vi "Test Pose.vi"() -> ()   [LabVIEW 2020, in "Rover.lvlib" / "Rover.lvclass"]
uses:
  Rover.lvclass
  Pose.ctl
  PID Tuning.ctl
  <vilib>/MakerHub/LINX/Public/Utilities/Open Local.vi
  <vilib>/MakerHub/LINX/LMH-LINX.lvlib
panel:
  out "OutR":i16(slide) scale=-32767.0..32767.0
  out "OutL":i16(slide) scale=-32767.0..32767.0
  out "Fault":bool
  in  "Turn":sgl(slide) scale=3.0..-3.0
  in  "Drive":sgl(slide) scale=-2.0..2.0
  in  "PID Tuning":T1
  out "XY Graph":cluster{"X":dbl, "Y":dbl}[](graph)
  out "Pose":T2
  in  "stop":bool
  out "error out":errorcluster
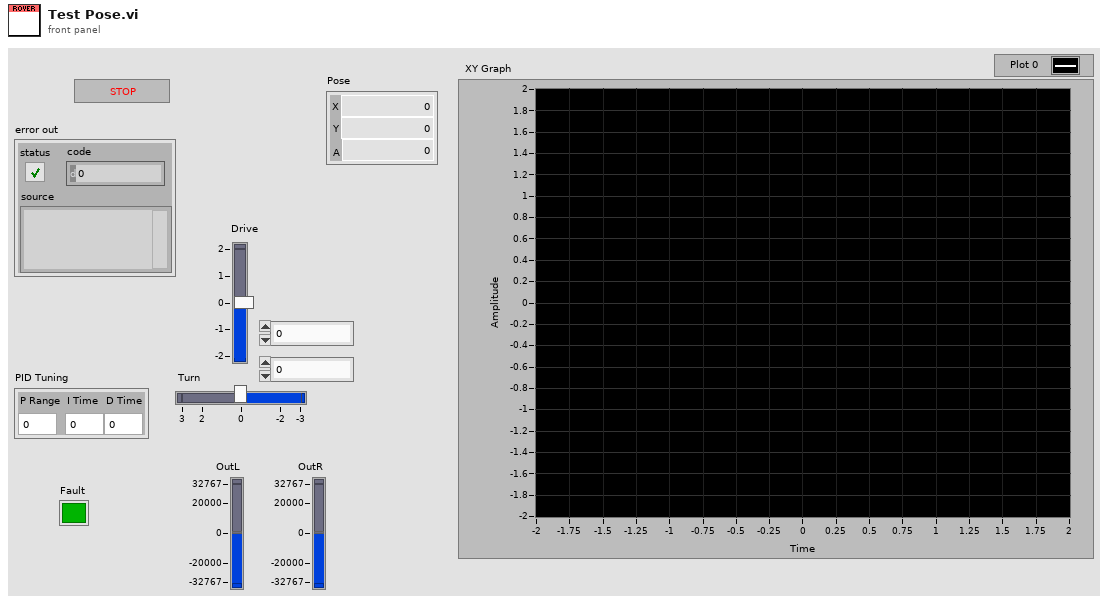
[diagram p1: front panel]
types:
  T1 = typedef "Rover.lvlib/Rover.lvclass/PID Tuning.ctl" = cluster{"P Range":sgl, "I Time":sgl, "D Time":sgl}
  T2 = typedef "Rover.lvlib/Rover.lvclass/Pose.ctl" = cluster{"X":sgl, "Y":sgl, "A":sgl}
  T3 = typedef "LMH-LINX.lvlib/LINX Ref.ctl" = cluster{"IO":T4, "Interface":T5, "LINX Device Config":T6}
  T4 = typedef "LMH-LINX.lvlib/Platform.ctl" = enum16{"Remote", "Local"}
  T5 = typedef "LMH-LINX.lvlib/Interface.ctl" = enum16{"Serial", "TCP"}
  T6 = typedef "LMH-LINX.lvlib/Device.lvlib/LINX Device Config.ctl" = cluster{"Interface":T5, "COM Port":refnum<visa-resource-name>, "TCP Configuration":T7, "Device Family":u8, "Device ID":u8, "Device Name":string, "TCP Ref":refnum<k5>, "Channels":T8}
  T7 = typedef "LMH-LINX.lvlib/Device.lvlib/TCP Config.ctl" = cluster{"IP Address":string, "Port":u16}
  T8 = typedef "LMH-LINX.lvlib/Channels.ctl" = cluster{"DI":u8[], "DO":u8[], "AI":u8[], "AO":u8[], "PWM":u8[], "QE":u8[], "UART":u8[], "I2C 2":u8[], "SPI":u8[], "CAN":u8[], "Servo":u8[], "AI Ref (V)":dbl, "AI Resolution (Bits)":u8, "AO Ref (V)":dbl, "AO Resolution (Bits)":u8}
  T9 = typedef "Rover.lvlib/Rover.lvclass/Outputs.ctl" = cluster{"Left":i16, "Right":i16}
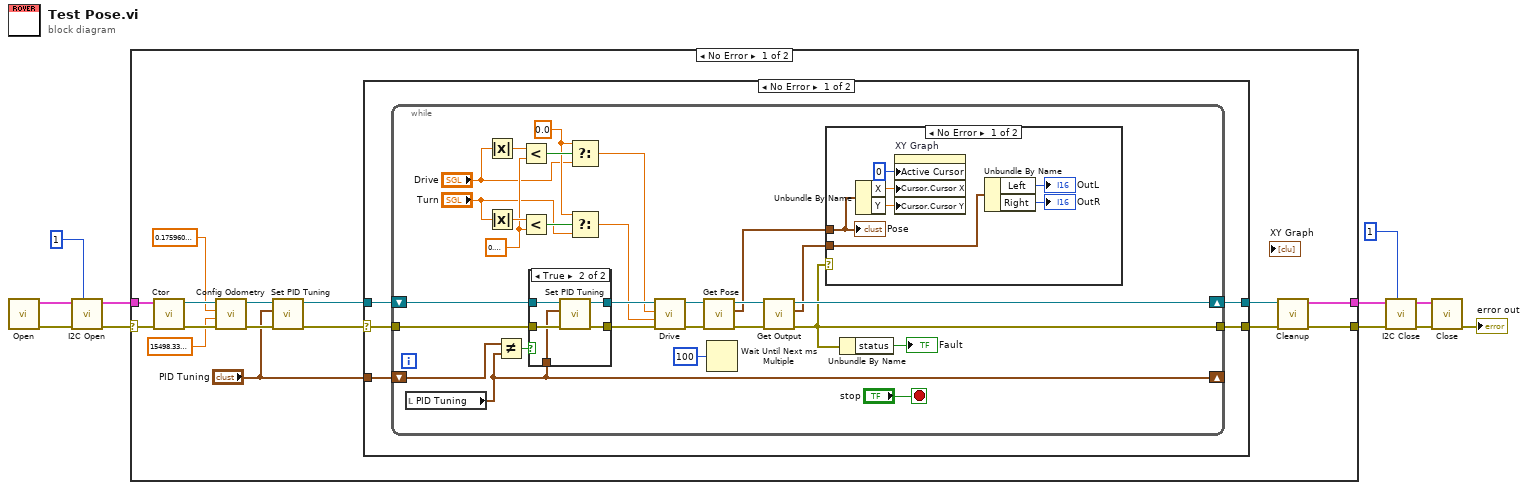
[diagram p0: block diagram]
diagram:
  n1 = call-poly <vilib>:"Open.vi"() -> ("Error Out"=w10:errorcluster, "LINX Resource"=w11:T3)  [unwired: 9 in, 1 out]
  n2 = call <vilib>:"I2C Open.vi"("I2C Channel (0)"=u8 1, "Error In"=w10, "LINX Resource"=w11) -> ("Error Out"=w9:errorcluster, "LINX Resource"=w8:T3)  [unwired: 7 in]
  n3 = case shown="No Error" w9 {
    selector: w9 -> [w25 w77]
    tunnel: w8 -> [w26 w76]
    tunnel: [w17 w77] -> w6
    tunnel: [w18 w76] -> w7
    frame No Error {
      n4 = call "Ctor.vi"("error in (no error)"=w25, "LINX Resource"=w26) -> ("error out"=w23:errorcluster, "Rover out"=w24:refnum<class "Rover.lvclass">)  [unwired: 8 in]
      n5 = call "Config Odometry.vi"("error in (no error)"=w23, "Ticks per Unit"=sgl 15498.331, "Wheel Width"=sgl 0.17596, "Rover in"=w24) -> ("error out"=w15:errorcluster, "Rover out"=w16:refnum<class "Rover.lvclass">)  [unwired: 6 in]
      n6 = call "Set PID Tuning.vi"("error in (no error)"=w15, "PID Tuning"="PID Tuning", "Rover in"=w16) -> ("error out"=w14:errorcluster, "Rover out"=w13:refnum<class "Rover.lvclass">)  [unwired: 7 in]
      n7 = case shown="No Error" w14 {
        selector: w14 -> [w30 w74]
        tunnel: w13 -> [w31 w75]
        tunnel: [w29 w75] -> w19
        tunnel: [w28 w74] -> w20
        tunnel: "PID Tuning" -> [w27 _]
        frame No Error {
          n8 = while {
            shift-right: [w46] -> w29
            shift-left: w31 -> [w53]
            shift-right: [w52] -> _
            shift-left: w27 -> [w56]
            tunnel: w30 -> [w54]
            tunnel: [w42] -> w28
            stop <- "stop" stop-if-true
            w36 = sgl 0.0 ("t")
            w39 = sgl 0.3 ("y")
            n9 = local read "PID Tuning"() -> (w52:T1)
            n10 = Absolute Value(x="Drive") -> (abs(x)=w41:sgl)
            n11 = Absolute Value(x="Turn") -> (abs(x)=w40:sgl)
            n12 = Not Equal?(x=w56, y=w52) -> (x != y?=w55:bool)
            n13 = Less?(x=w41, y=w39) -> (x < y?=w38:bool)
            n14 = Less?(x=w40, y=w39) -> (x < y?=w37:bool)
            n15 = case shown="True" w55 {
              tunnel: w54 -> [w67 w72]
              tunnel: w53 -> [w68 w73]
              tunnel: [w68 w69] -> w51
              tunnel: [w67 w70] -> w50
              tunnel: w52 -> [_ w71]
              frame False {
              }
              frame True {
                n16 = call "Set PID Tuning.vi"("error in (no error)"=w72, "PID Tuning"=w71, "Rover in"=w73) -> ("error out"=w70:errorcluster, "Rover out"=w69:refnum<class "Rover.lvclass">)  [unwired: 7 in]
              }
            }
            n17 = Select(t=w36, s=w38, f="Drive") -> (s? t:f=w32:sgl)
            n18 = Select(t=w36, s=w37, f="Turn") -> (s? t:f=w33:sgl)
            n19 = call "Drive.vi"("error in (no error)"=w50, "Turn"=w33, "Drive"=w32, "Rover in"=w51) -> ("error out"=w49:errorcluster, "Rover out"=w48:refnum<class "Rover.lvclass">)  [unwired: 6 in]
            n20 = call "Get Pose.vi"("error in (no error)"=w49, "Rover in"=w48) -> ("error out"=w57:errorcluster, "Pose"=w44:T2, "Rover out"=w58:refnum<class "Rover.lvclass">)  [unwired: 7 in]
            n21 = Wait Until Next ms Multiple(millisecond multiple=u32 100) -> ()  [unwired: 1 out]
            n22 = call "Get Output.vi"("error in (no error)"=w57, "Rover in"=w58) -> ("error out"=w42:errorcluster, "Outputs"=w43:T9, "Rover out"=w46:refnum<class "Rover.lvclass">)  [unwired: 7 in]
            n23 = case shown="No Error" w42 {
              tunnel: w44 -> [w61 _]
              tunnel: w43 -> [w60 _]
              frame No Error {
                n24 = Unbundle By Name(w61) -> ("X"=w66:sgl, "Y"=w65:sgl)
                n25 = property on="XY Graph" class="XYGraph (strict)"("Active Cursor"=u32 0, "Cursor.Cursor X"=w66, "Cursor.Cursor Y"=w65) -> ()  [unwired: 2 in, 2 out]
                n26 = Unbundle By Name(w60) -> ("Left"=→"OutL":i16, "Right"=→"OutR":i16)
                "Pose" <- w61
              }
              frame Error {
              }
            }
            n27 = Unbundle By Name(w42) -> ("status"=→"Fault":bool)
          }
        }
        frame Error {
        }
      }
      n28 = call "Cleanup.vi"("error in (no error)"=w20, "Rover in"=w19) -> ("error out"=w17:errorcluster, "LINX Resource"=w18:T3)  [unwired: 8 in]
    }
    frame Error {
    }
  }
  n29 = call <vilib>:"I2C Close.vi"("I2C Channel (0)"=u8 1, "Error In"=w6, "LINX Resource"=w7) -> ("Error Out"=w3:errorcluster, "LINX Resource"=w4:T3)  [unwired: 7 in]
  n30 = call <vilib>:"Close.vi"("Error In"=w3, "LINX Resource"=w4) -> ("Error Out"=→"error out":errorcluster)  [unwired: 9 in]
